vi "PincerCtrl v2.vi"(8 "error in":errorcluster, 9 "Duty Limits [max,min]":dbl[](array[numeric])=[0.06, 0.05], 10 "Motion [%]":dbl, 11 "FPGA VI Reference In":refnum<k20>) -> (0 "error out":errorcluster, 3 "FPGA VI Reference Out":refnum<k20>)   [LabVIEW 2010]
uses:
  <vilib>/rvi/interface/nirviReadWriteControl/nirviReadWriteControl.xnode
  FPGA Bitfiles/IRISSControl_FPGATarget_IRISSFPGAIOv3.3_r-h2UkgnQFc.lvbitx
  IRISS_FPGA_IO_v3.3.vi
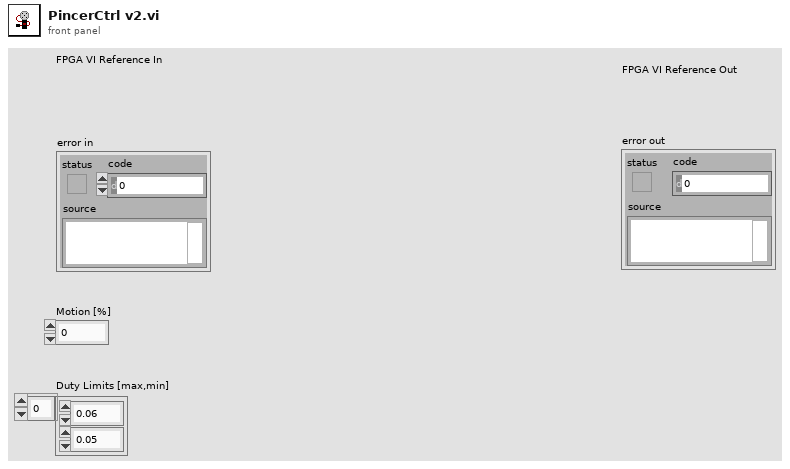
[diagram p1: front panel]
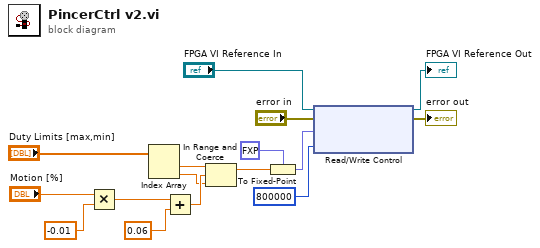
[diagram p0: block diagram]
diagram:
  n1 = Multiply(x="Motion [%]", y=-0.01) -> (x*y=w9:dbl)
  n2 = Index Array(array="Duty Limits [max,min]") -> (element #1=w5:dbl, element #2=w4:dbl)  [unwired: 2 in]
  n3 = Add(x=w9, y=0.06) -> (x+y=w7:dbl)
  n4 = In Range and Coerce(upper limit=w5, x=w7, lower limit=w4) -> (coerced(x)=w3:dbl)  [unwired: 1 out]
  n5 = To Fixed-Point(fixed-point type=fxp<+,32,0> 0.0 ("PWM1"), number=w3) -> (fixed-point=w1:fxp<+,32,0>)
  n6 = xnode "Read/Write Control"("FPGA VI Reference In"="FPGA VI Reference In", "error in"="error in", "PWM1"=w1, "Period 1 (Ticks)"=u32 800000) -> ("FPGA VI Reference Out"=→"FPGA VI Reference Out":refnum<k20>, "error out"=→"error out":errorcluster)
